vi "tearDown.vi"(8 "error in (no error)":errorcluster, 11 "reference in":refnum<class "NI-SWITCH Messaging Tests.lvclass">) -> (0 "error out":errorcluster, 3 "reference out":refnum<class "NI-SWITCH Messaging Tests.lvclass">)   [LabVIEW 2017, in "NI-SWITCH Messaging Tests.lvclass"]
doc: "tearDown runs after the test method has completed. Use this method to clean up any operations or references that were opened by setUp or the test method. Unit tests should be independent of other unit tests so this VI should ensure that the next test can run in a 'clean' test environment."
uses:
  NI-SWITCH Messaging Tests.lvclass
  NI-SWITCH Messaging Tests.lvclass/NI-SWITCH Messaging Tests.ctl
  Includes/CDMessaging.lvlibp/Producer/Abstract Producer/Abstract Producer.lvclass
  Includes/CDMessaging.lvlibp/Consumer/Abstract Consumer/Abstract Consumer.lvclass
  Includes/CDMessaging.lvlibp/Switch/Abstract Switch Consumer/Abstract Switch Consumer.lvclass
  C:/Dev/GitHub/niveristand-slsc-switch-message-library/Includes/CDMessaging.lvlibp/Consumer/Abstract Consumer/Abstract Consumer.lvclass
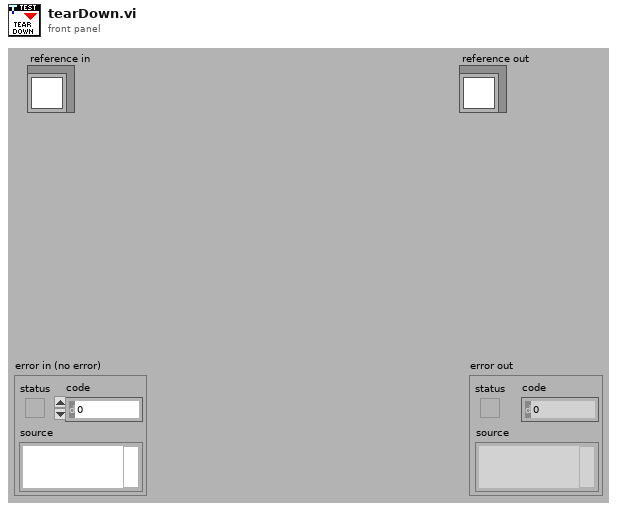
[diagram p1: front panel]
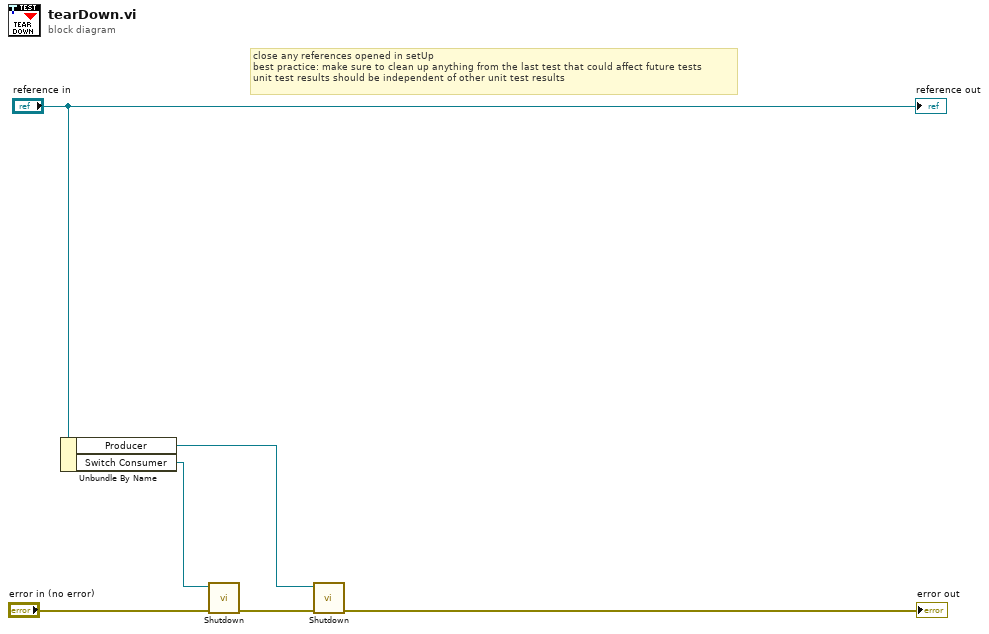
[diagram p0: block diagram]
diagram:
  # "close any references opened in setUp\nbest practice: make sure to clean up anything from the last test that could affect future tests\nunit test results should be independent of other unit test results"
  n1 = Unbundle By Name("reference in") -> ("Producer"=w1:refnum<class "Abstract Producer.lvclass">, "Switch Consumer"=w2:refnum<class "Abstract Switch Consumer.lvclass">)
  n2 = call "Shutdown.vi"("error in (no error)"="error in (no error)", "Abstract Consumer in"=w2) -> ("error out"=w4:errorcluster)  [unwired: 8 in, 1 out]
  n3 = call "Shutdown.vi"("error in (no error)"=w4, "Abstract Producer in"=w1) -> ("error out"=→"error out":errorcluster)  [unwired: 8 in, 1 out]
  "reference out" <- "reference in"
